vi "sub filt array by tag.vi"(8 "error in":errorcluster, 10 "tag":string, 11 "string array":string[](array[string])) -> (0 "error out":errorcluster, 3 "filted string array":string[](array[string]))   [LabVIEW 2018, in "Frame Analizer.lvclass"]
uses:
  Frame Analizer.lvclass
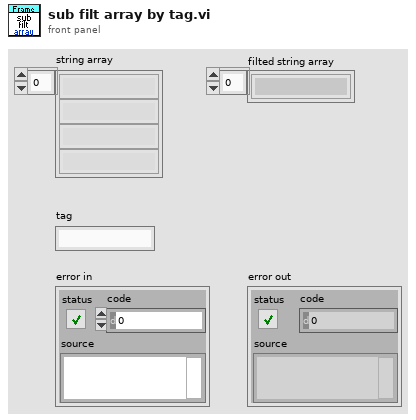
[diagram p1: front panel]
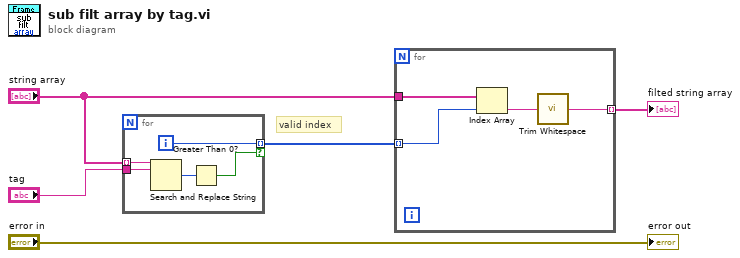
[diagram p0: block diagram]
diagram:
  # "valid index"
  n1 = for {
    tunnel: "string array" -> [w10] mode=indexing
    tunnel: "tag" -> [w9]
    tunnel: [w6] -> w4 mode=indexing if=w7
    i -> [w6]
    n2 = Search and Replace String(input string=w10, search string=w9) -> (number of replacements=w8:i32)  [unwired: 6 in, 3 out]
    n3 = Greater Than 0?(x=w8) -> (x > 0?=w7:bool)
  }
  n4 = for {
    tunnel: w4 -> [w13] mode=indexing
    tunnel: "string array" -> [w14]
    tunnel: [w11] -> w2 mode=indexing
    n5 = Index Array(array=w14, index=w13) -> (element=w12:string)
    n6 = call <vilib>:"Trim Whitespace.vi"("string"=w12) -> ("trimmed string"=w11:string)  [unwired: 1 in]
  }
  "filted string array" <- w2
  "error out" <- "error in"
